vi "relatorio.vi"   [LabVIEW 2016]
uses:
  <vilib>/addons/_office/excel.llb/Excel Easy Table (str).vi
  <vilib>/Utility/NIReport.llb/NI_report.lvclass
  <vilib>/addons/_office/NI_ReportGenerationToolkit.lvlib
types:
  T1 = enum16{"Standard Report", "HTML", "Word", "Excel"}
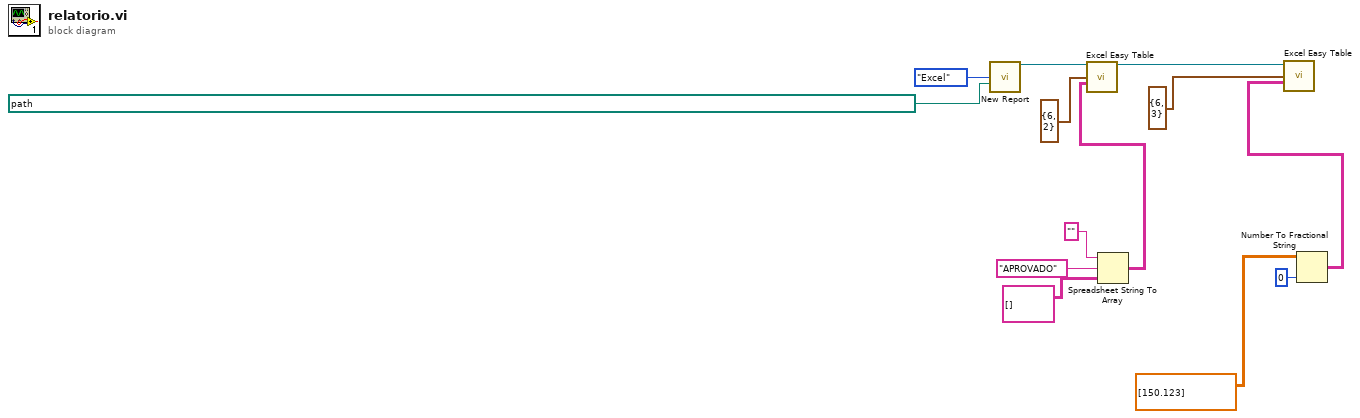
[diagram p0: block diagram]
diagram:
  n1 = call <vilib>:"New Report.vi"("report type"=T1."Excel", "template (empty)"=path "D:/UFSM/Engenharia de Controle e Automação/8 Semestre/Projeto Integrador - DPEE 1064/LabVIEW/Projeto Integrador - William Rocha/relatorio/Bateria Unipower 1.xlsx") -> ("report out"=w6:refnum<class "NI_report.lvclass">)  [unwired: 12 in, 1 out]
  n2 = Spreadsheet String To Array(format string="", spreadsheet string="APROVADO", array type (2D Dbl)=string[][] []) -> (array=w8:string[][])  [unwired: 1 in]
  n3 = call-poly <vilib>:"Excel Easy Table.vi"("report in"=w6, "start (0, 0)"=cluster{"row":i32, "column":i32} {"row"=6, "column"=2}, "text data"=w8) -> ("report out"=w4:refnum<class "NI_report.lvclass">)  [unwired: 8 in, 4 out]
  n4 = Number To Fractional String(number=dbl[][] [[150.123]], precision (6)=i16 0) -> (F-format string=w1:string[][])  [unwired: 2 in]
  n5 = call-poly <vilib>:"Excel Easy Table.vi"("report in"=w4, "start (0, 0)"=cluster{"row":i32, "column":i32} {"row"=6, "column"=3}, "text data"=w1) -> ()  [unwired: 8 in, 5 out]
